vi "DiametroRondelle.vi"() -> ()   [LabVIEW 2020]
panel:
  out "Array 2":dbl[](array[numeric])
  out "Array":dbl[](array[numeric])
  in  "Calibration Image":path=path "C:/Users/Dell/Desktop/Esame/LOAD/CalibrazioneMisura/calib-info.png"
  out "Image":T1(plugin-control)
  in  "error in (no error)":errorcluster
  in  "Image Path":path=path "C:/Users/Dell/Desktop/Esame/LOAD/CalibrazioneMisura/Piastra3.png"
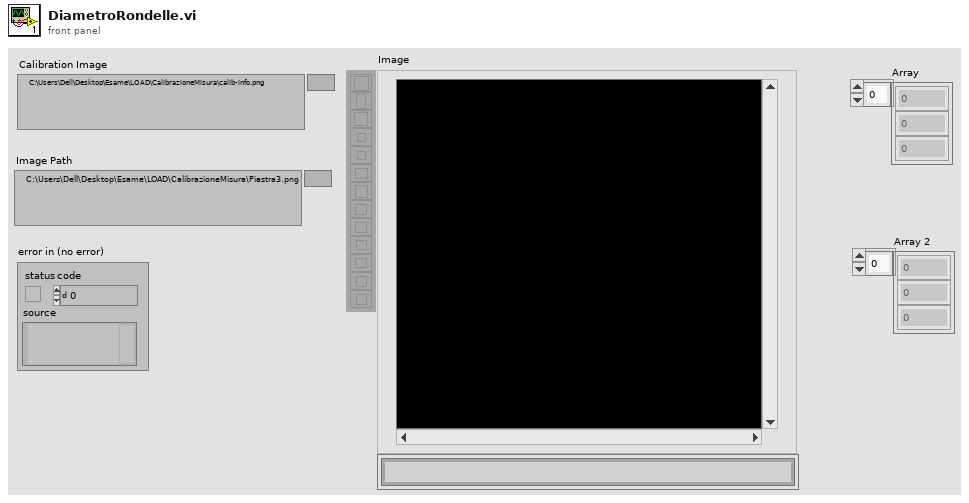
[diagram p1: front panel]
types:
  T1 = typedef "IMAQ Image.ctl" = refnum<image>
  T2 = typedef "Edge New.ctl" = cluster{"Location (Pixel)":cluster{"X":sgl, "Y":sgl}, "Location (Real-World)":cluster{"X":sgl, "Y":sgl}, "Distance (Pixel)":dbl, "Distance (Real-World)":dbl, "Strength":dbl, "Noise":dbl, "Rising?":bool}
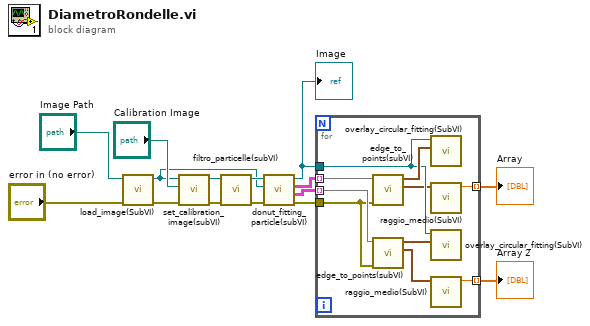
[diagram p0: block diagram]
diagram:
  n1 = call "load_image(SubVI).vi"("error in (no error)"="error in (no error)", "Image Path"="Image Path") -> ("error out"=w7:errorcluster, "Image GRAY"=w1:T1)  [unwired: 7 in, 1 out]
  n2 = call "set_calibration_image(subVI).vi"("error in (no error)"=w7, "File Path"="Calibration Image", "Image Dst"=w1) -> ("error out"=w8:errorcluster, "Image Out"=w9:T1)  [unwired: 6 in, 1 out]
  n3 = call "filtro_particelle(subVI).vi"("error in (no error)"=w8, "Image Src"=w9) -> ("error out"=w12:errorcluster, "Image"=w13:T1)  [unwired: 8 in]
  n4 = call "donut_fitting_particle(subVI).vi"("error in (no error)"=w12, "Image Dst"=w1, "Image Src"=w13) -> ("error out"=w5:errorcluster, "First Edges"=w6:T2[][], "Last Edges"=w11:T2[][], "Image"=w4:T1)  [unwired: 5 in]
  "Image" <- w4
  n5 = for {
    tunnel: w11 -> [w25] mode=indexing
    tunnel: w6 -> [w24] mode=indexing
    tunnel: w5 -> [w23]
    tunnel: w4 -> [w21]
    tunnel: [w17] -> w3 mode=indexing
    tunnel: [w16] -> w2 mode=indexing
    n6 = call "edge_to_points(subVI).vi"("error in (no error)"=w23, "First Edges"=w25) -> ("points (real-world)"=w19:cluster{"X":sgl, "Y":sgl}[], "points (pixel)"=w22:cluster{"X":sgl, "Y":sgl}[])  [unwired: 7 in, 1 out]
    n7 = call "edge_to_points(subVI).vi"("error in (no error)"=w23, "First Edges"=w24) -> ("points (real-world)"=w18:cluster{"X":sgl, "Y":sgl}[], "points (pixel)"=w20:cluster{"X":sgl, "Y":sgl}[])  [unwired: 7 in, 1 out]
    n8 = call "overlay_circular_fitting(SubVI).vi"("points (pixel)"=w22, "image dest"=w21) -> ()  [unwired: 7 in, 3 out]
    n9 = call "raggio_medio(SubVI).vi"("Radial Points"=w19) -> ("Radius"=w17:dbl)  [unwired: 9 in, 1 out]
    n10 = call "overlay_circular_fitting(SubVI).vi"("points (pixel)"=w20, "image dest"=w21) -> ()  [unwired: 7 in, 3 out]
    n11 = call "raggio_medio(SubVI).vi"("Radial Points"=w18) -> ("Radius"=w16:dbl)  [unwired: 9 in, 1 out]
  }
  "Array" <- w3
  "Array 2" <- w2
